vi "test_Basic Deployment.vi"(8 "error in (no error)":errorcluster, 11 "TestCase in":refnum<class "TLCD System Tests.lvclass">) -> (0 "error out":errorcluster, 3 "TestCase out":refnum<class "TLCD System Tests.lvclass">)   [LabVIEW 2019, in "TLCD System Tests.lvclass"]
uses:
  TLCD System Tests.lvclass
  <vilib>/addons/_JKI Toolkits/VI Tester/TestCase.llb/TestCase.lvclass
  TLCD Test Class/TLCD Test Class.lvclass
  <vilib>/WebDAVClient/NI_WebDAV.lvlib
  C:/Program Files (x86)/National Instruments/LabVIEW 2019/vi.lib/addons/_JKI Toolkits/VI Tester/TestCase.llb/TestCase.lvclass
panel:
  out "Log Exists ?":bool
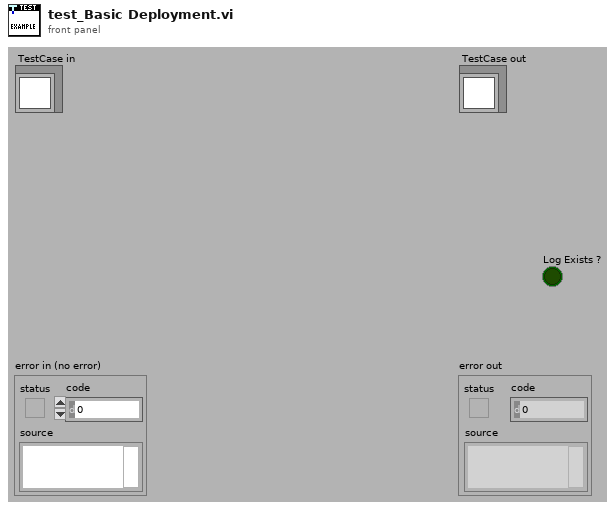
[diagram p1: front panel]
types:
  T1 = typedef "NI_WebDAV.lvlib/SessionHandle.ctl" = refnum<k1>
  T2 = typedef "NI_WebDAV.lvlib/FileInfo.ctl" = cluster{"type":string, "size":u64, "last modification":timestamp, "display name":string, "uri":string}
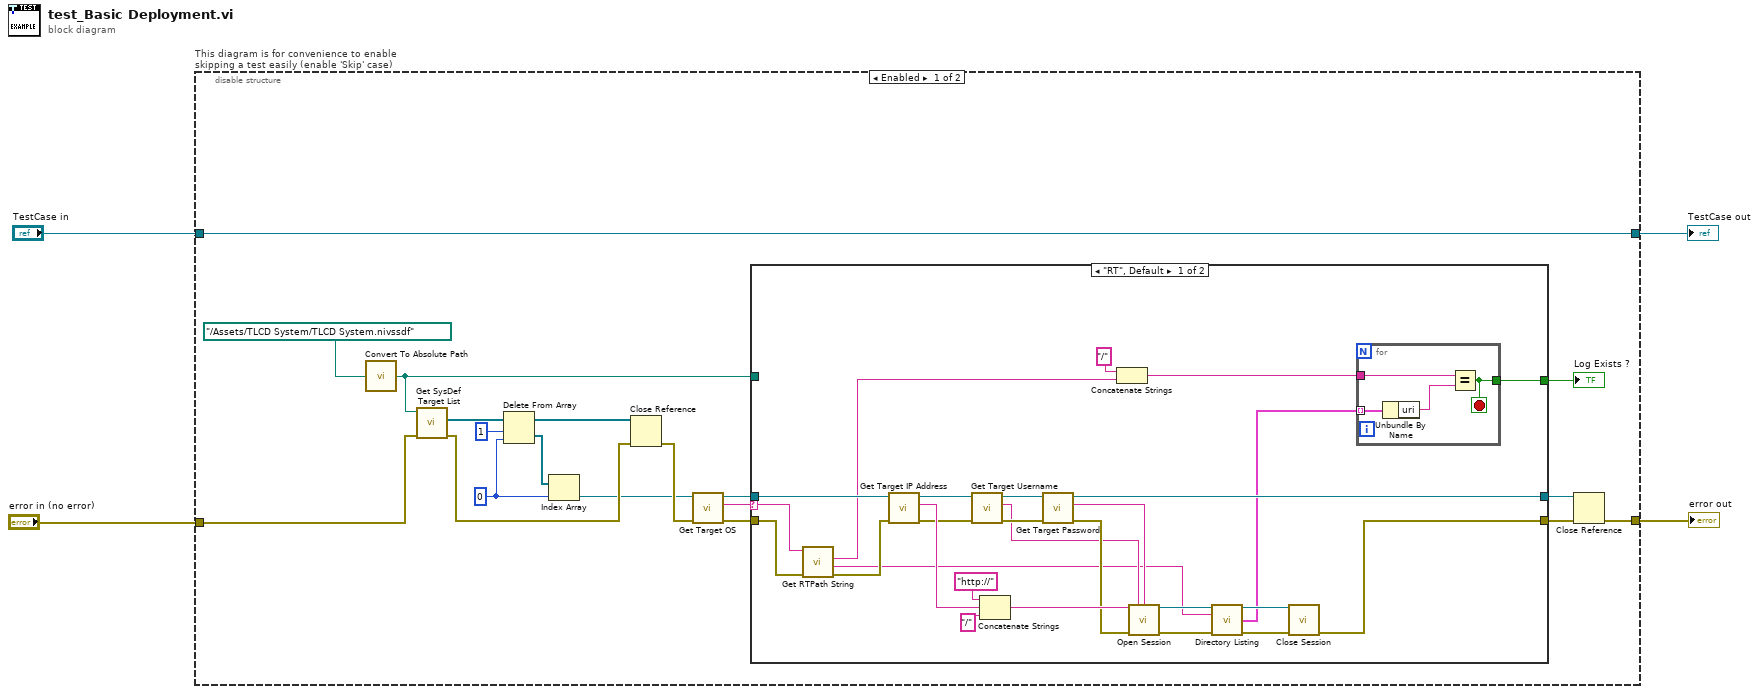
[diagram p0: block diagram]
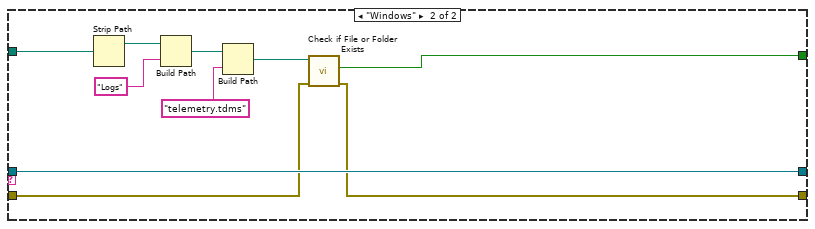
[diagram p2: hidden frame]
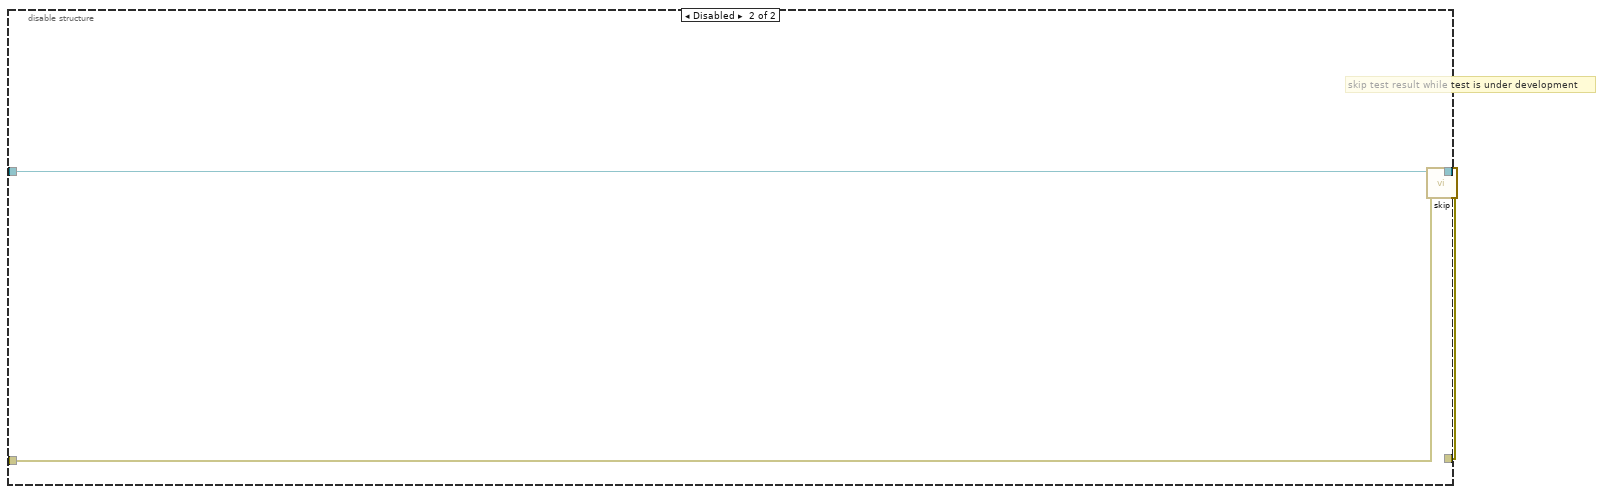
[diagram p3: hidden frame]
diagram:
  n1 = disable-structure "This diagram is for convenience to enable skipping a test easily (enable 'Skip' case)" shown="Enabled" {
    disable-tunnel: "TestCase in" -> [w23 w68]
    disable-tunnel: [w23 w66] -> w1
    disable-tunnel: [w20 w67] -> w3
    disable-tunnel: "error in (no error)" -> [w21 w65]
    frame Enabled {
      w16 = 0 ("index")
      n2 = call "Convert To Absolute Path.vi"("System Definition File Path"=path "../Assets/TLCD System/TLCD System.nivssdf" ("relative base path")) -> ("Absolute path"=w6:path)
      n3 = call "Get SysDef Target List.vi"("error in (no error)"=w21, "System Definition Path"=w6) -> ("error out"=w14:errorcluster, "Target List"=w19:refnum<k24>[])  [unwired: 8 in]
      n4 = Delete From Array(array=w19, length=1, index=w16) -> (deleted portion=w17:refnum<k24>[], array with subset deleted=w15:refnum<k24>[])
      n5 = Index Array(array=w17, index=w16) -> (element=w10:refnum<k24>)
      n6 = Close Reference(reference=w15, error in (no error)=w14) -> (error out=w11:errorcluster)
      n7 = call "Get Target OS.vi"("error in (no error)"=w11, "Target ref in"=w10) -> ("error out"=w9:errorcluster, "OperatingSystem"=w7:string, "Target ref out"=w8:refnum<k24>)  [unwired: 7 in]
      n8 = case shown="\"RT\", Default" w7 {
        selector: w7 -> [w50 _]
        tunnel: [w32 w56] -> w13
        tunnel: [w33 w64] -> w12
        tunnel: w9 -> [w49 w57]
        tunnel: w8 -> [w48 w64]
        tunnel: w6 -> [_ w63]
        tunnel: [w24 w55] -> w5
        frame "RT", Default {
          n9 = call "Get RTPath String.vi"("error in (no error)"=w49, "Target OS in"=w50) -> ("error out"=w47:errorcluster, "RT Folder Path"=w29:string, "RT File Path"=w27:string)  [unwired: 6 in, 1 out]
          n10 = call "Get Target IP Address.vi"("error in (no error)"=w47, "Target ref in"=w48) -> ("error out"=w40:errorcluster, "IPAddress"=w45:string, "Target ref out"=w42:refnum<k24>)  [unwired: 7 in]
          n11 = call "Get Target Username.vi"("error in (no error)"=w40, "Target ref in"=w42) -> ("error out"=w39:errorcluster, "Username"=w36:string, "Target ref out"=w41:refnum<k24>)  [unwired: 7 in]
          n12 = Concatenate Strings("http://" ("string"), w45, "/" ("string")) -> (w43:string)
          n13 = call "Get Target Password.vi"("error in (no error)"=w39, "Target ref in"=w41) -> ("error out"=w38:errorcluster, "Password"=w37:string, "Target ref out"=w33:refnum<k24>)  [unwired: 7 in]
          n14 = Concatenate Strings("/" ("string"), w27) -> (w26:string)
          n15 = call <vilib>:"Open Session.vi"("host uri prefix"=w43, "username"=w36, "password"=w37, "error in (no error)"=w38) -> ("session handle out"=w34:T1, "error out"=w35:errorcluster)  [unwired: 10 in]
          n16 = call <vilib>:"Directory Listing.vi"("session handle"=w34, "relative uri"=w29, "error in (no error)"=w35) -> ("session handle out"=w31:T1, "file list"=w28:T2[], "error out"=w30:errorcluster)  [unwired: 9 in, 1 out]
          n17 = call <vilib>:"Close Session.vi"("session handle"=w31, "error in (no error)"=w30) -> ("error out"=w32:errorcluster)  [unwired: 13 in]
          n18 = for {
            tunnel: w28 -> [w54] mode=indexing
            tunnel: w26 -> [w52]
            tunnel: [w51] -> w24
            stop <- w51 stop-if-true
            n19 = Unbundle By Name(w54) -> ("uri"=w53:string)
            n20 = Equal?(x=w52, y=w53) -> (x = y?=w51:bool)
          }
        }
        frame "Windows" {
          n21 = Strip Path(path=w63) -> (stripped path=w62:path)  [unwired: 1 out]
          n22 = Build Path(base path=w62, name or relative path="Logs") -> (appended path=w60:path)
          n23 = Build Path(base path=w60, name or relative path="telemetry.tdms") -> (appended path=w58:path)
          n24 = call <vilib>:"Check if File or Folder Exists.vi"("error in (no error)"=w57, "path"=w58) -> ("error out"=w56:errorcluster, "file or folder exists?"=w55:bool)  [unwired: 7 in, 1 out]
        }
      }
      "Log Exists ?" <- w5
      n25 = Close Reference(reference=w12, error in (no error)=w13) -> (error out=w20:errorcluster)
    }
    frame Disabled {
      # "skip test result while test is under development"
      n26 = call <vilib>:"skip.vi"("error in (no error)"=w65, "TestCase in"=w68) -> ("error out"=w67:errorcluster, "TestCase out"=w66:refnum<class "TLCD System Tests.lvclass">)  [unwired: 8 in]
    }
  }
  "error out" <- w3
  "TestCase out" <- w1
